vi "Configure Data Log.vi"(4 "Data Log Offset (0.0)":dbl format="%^.3e", 5 "Data Log Duration (30 s)":i32=30, 6 "Data Log Period (0.1 s)":dbl=0.1 format="%^.3e", 7 "Enable Data Log (True)":bool=TRUE, 8 "error in (no error)":errorcluster {"code" format="%.0x"}, 9 "Data Log Type (1: Voltage)":i32(ring)=1 items=["Voltage"=1, "Current"=0], 10 "Channel Name (1)":string="1", 11 "VISA resource name":refnum<visa-resource-name>) -> (0 "error out":errorcluster {"code" format="%.0x"}, 3 "VISA resource name out":refnum<visa-resource-name>)   [LabVIEW 2018, in "Agilent N6700 Series.lvlib"]
doc: "Configures the data log type, duration, period, offset and sets the state of the data log.\n\n<b>Note:</b>\nThis VI only applies to the N6705B and N6705C DC Power Analyzer."
uses:
  Agilent N6700 Series.lvlib
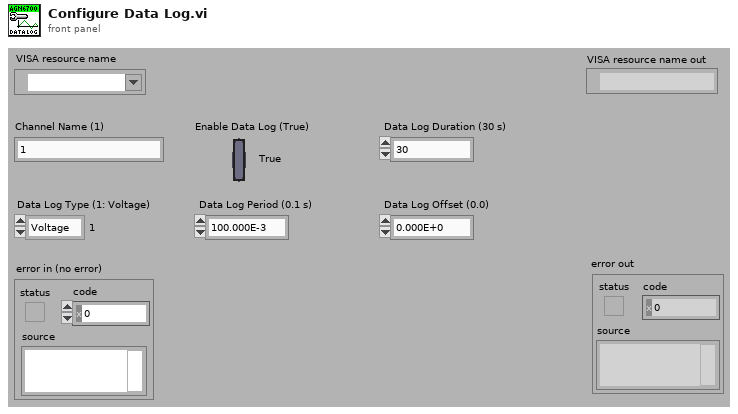
[diagram p1: front panel]
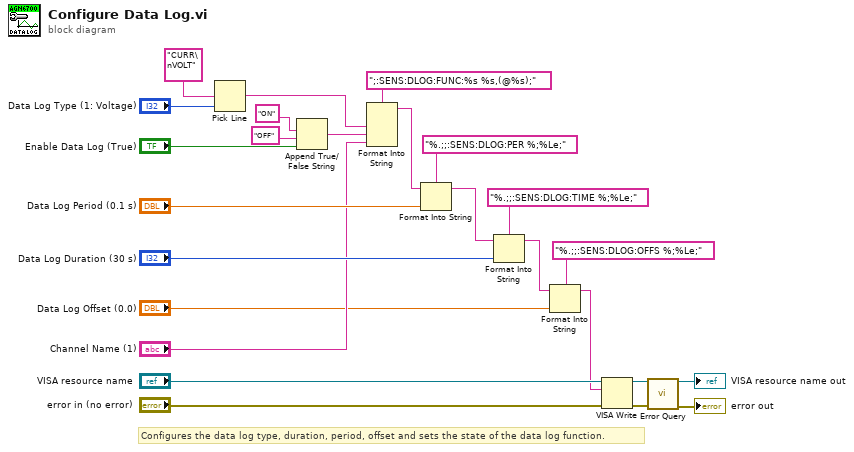
[diagram p0: block diagram]
diagram:
  # "Configures the data log type, duration, period, offset and sets the state of the data log function."
  n1 = Pick Line(multi-line string="CURR\nVOLT", line index="Data Log Type (1: Voltage)") -> (output string=w9:string)  [unwired: 1 in]
  n2 = Append True/False String(1:"Enable Data Log (True)", 2:"OFF", 3:"ON") -> (0:w8:string)  [unwired: 1 in]
  n3 = Format Into String(format string=";:SENS:DLOG:FUNC:%s %s,(@%s);", w9, w8, "Channel Name (1)") -> (resulting string=w6:string)  [unwired: 2 in, 1 out]
  n4 = Format Into String(format string="%.;;:SENS:DLOG:PER %;%Le;", initial string=w6, "Data Log Period (0.1 s)") -> (resulting string=w19:string)  [unwired: 1 in, 1 out]
  n5 = Format Into String(format string="%.;;:SENS:DLOG:TIME %;%Le;", initial string=w19, "Data Log Duration (30 s)") -> (resulting string=w3:string)  [unwired: 1 in, 1 out]
  n6 = Format Into String(format string="%.;;:SENS:DLOG:OFFS %;%Le;", initial string=w3, "Data Log Offset (0.0)") -> (resulting string=w2:string)  [unwired: 1 in, 1 out]
  n7 = VISA Write(VISA resource name="VISA resource name", write buffer=w2, error in (no error)="error in (no error)") -> (VISA resource name out=w21:refnum<visa-resource-name>, error out=w20:errorcluster)  [unwired: 1 out]
  n8 = call "Error Query.vi"("VISA resource name"=w21, "error in (no error)"=w20) -> ("VISA resource name out"=→"VISA resource name out":refnum<visa-resource-name>, "error out"=→"error out":errorcluster)  [unwired: 10 in, 2 out]
